vi "UNDTClasterToTbl.vi"(11 "UNDT_Cluster":T1 {"Gain Coeff" format="%#_6e"; "Reserve 1" format="%02x"; "Mux TX/RX" format="%02x"; "ScanDelay" format="%02x"; "PacketCounter" format="%08x"; "SamplingInterval" format="%#_6e"; "Lose Packet" format="%08x"; "EncodersParam2" format="%016x"; "EncodersParam1" format="%016x"; "CRC 8" format="%02x"; "N chanel" format="%02x"; "N tick" format="%02x"; "Ncycle" format="%04x"; "FrameFormatVersion" format="%02x"; "MagicWord" format="%.0x"}) -> (2 "appended array":string[](array[string]), 3 "Table Control":string[][](table))   [LabVIEW 2017]
uses:
  Control_EU/UNDT_ClusterPackRevers (Type).ctl
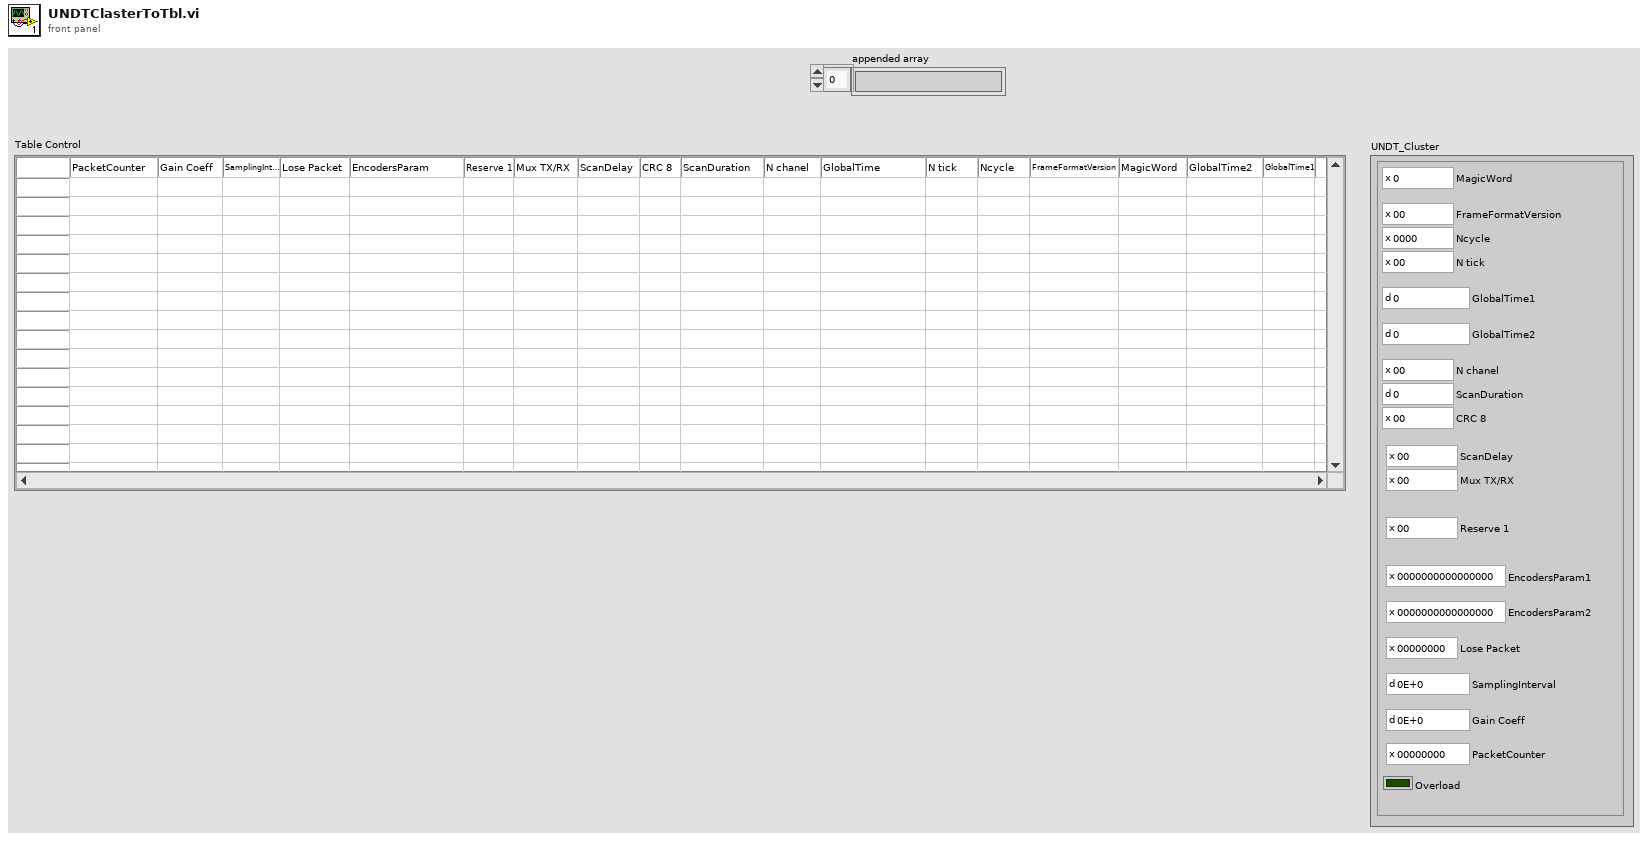
[diagram p1: front panel]
types:
  T1 = typedef "UNDT_ClusterPackRevers (Type).ctl" = cluster{"PacketCounter":u32, "Gain Coeff":sgl, "SamplingInterval":sgl, "Lose Packet":u32, "EncodersParam2":u64, "EncodersParam1":u64, "Reserve 1":u8, "Mux TX/RX":u8, "ScanDelay":u16, "CRC 8":u8, "ScanDuration":u16, "N chanel":u8, "GlobalTime2":u32, "GlobalTime1":u32, "N tick":u8, "Ncycle":u16, "FrameFormatVersion":u8, "MagicWord":u32, "Overload":bool}
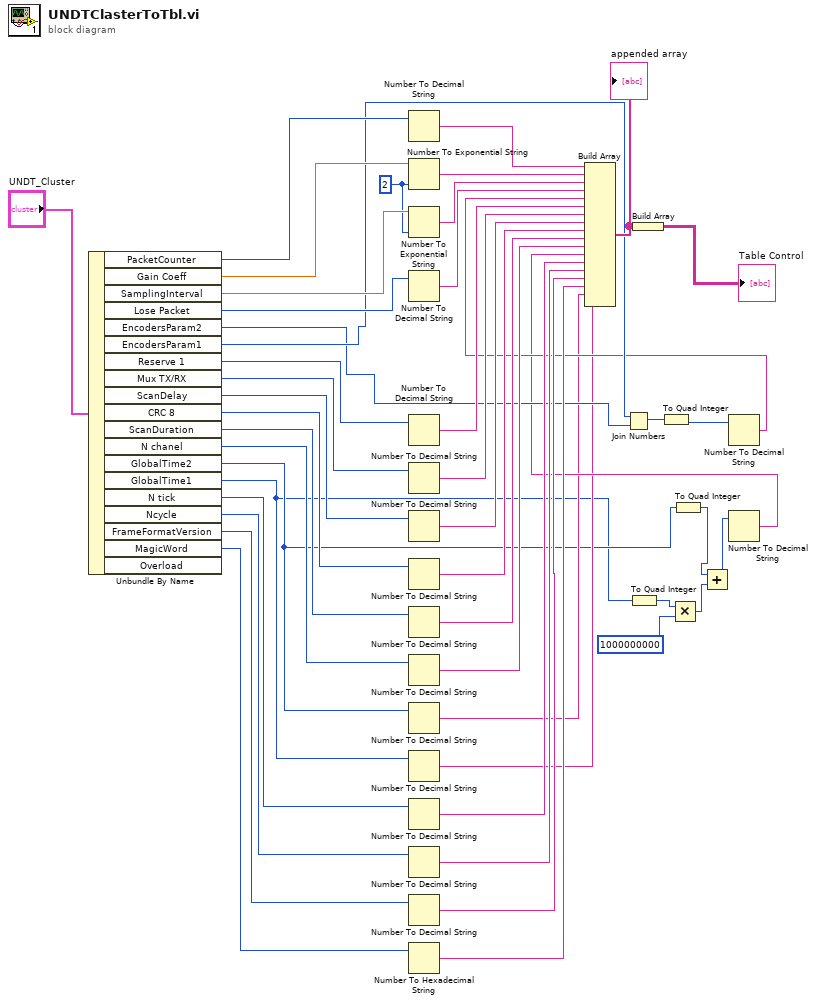
[diagram p0: block diagram]
diagram:
  w16 = i16 2 ("precision (6)")
  n1 = Unbundle By Name("UNDT_Cluster") -> ("PacketCounter"=w46:u32, "Gain Coeff"=w35:sgl, "SamplingInterval"=w19:sgl, "Lose Packet"=w18:u32, "EncodersParam2"=w14:u64, "EncodersParam1"=w15:u64, "Reserve 1"=w45:u8, "Mux TX/RX"=w44:u8, "ScanDelay"=w43:u16, "CRC 8"=w42:u8, "ScanDuration"=w41:u16, "N chanel"=w40:u8, "GlobalTime2"=w2:u32, "GlobalTime1"=w1:u32, "N tick"=w39:u8, "Ncycle"=w38:u16, "FrameFormatVersion"=w37:u8, "MagicWord"=w36:u32)  [unwired: 1 out]
  n2 = Number To Decimal String(number=w46) -> (decimal integer string=w34:string)  [unwired: 1 in]
  n3 = Number To Exponential String(number=w35, precision (6)=w16) -> (E-format string=w33:string)  [unwired: 2 in]
  n4 = Number To Exponential String(number=w19, precision (6)=w16) -> (E-format string=w32:string)  [unwired: 2 in]
  n5 = Number To Decimal String(number=w18) -> (decimal integer string=w17:string)  [unwired: 1 in]
  n6 = Number To Decimal String(number=w45) -> (decimal integer string=w31:string)  [unwired: 1 in]
  n7 = Number To Decimal String(number=w44) -> (decimal integer string=w30:string)  [unwired: 1 in]
  n8 = Number To Decimal String(number=w43) -> (decimal integer string=w29:string)  [unwired: 1 in]
  n9 = Number To Decimal String(number=w42) -> (decimal integer string=w28:string)  [unwired: 1 in]
  n10 = Number To Decimal String(number=w41) -> (decimal integer string=w27:string)  [unwired: 1 in]
  n11 = Number To Decimal String(number=w40) -> (decimal integer string=w26:string)  [unwired: 1 in]
  n12 = Number To Decimal String(number=w2) -> (decimal integer string=w9:string)  [unwired: 1 in]
  n13 = Number To Decimal String(number=w1) -> (decimal integer string=w8:string)  [unwired: 1 in]
  n14 = Number To Decimal String(number=w39) -> (decimal integer string=w25:string)  [unwired: 1 in]
  n15 = Number To Decimal String(number=w38) -> (decimal integer string=w24:string)  [unwired: 1 in]
  n16 = Number To Decimal String(number=w37) -> (decimal integer string=w23:string)  [unwired: 1 in]
  n17 = Number To Hexadecimal String(2:w36) -> (0:w22:string)  [unwired: 1 in]
  n18 = Join Numbers(hi=w15, lo=w14) -> ((hi.lo)=w13:u64)
  n19 = To Quad Integer(1:w1) -> (0:w7:i64)
  n20 = To Quad Integer(1:w13) -> (0:w12:i64)
  n21 = Multiply(x=w7, y=i64 1000000000) -> (x*y=w5:i64)
  n22 = To Quad Integer(1:w2) -> (0:w4:i64)
  n23 = Add(x=w4, y=w5) -> (x+y=w3:i64)
  n24 = Number To Decimal String(number=w12) -> (decimal integer string=w11:string)  [unwired: 1 in]
  n25 = Number To Decimal String(number=w3) -> (decimal integer string=w10:string)  [unwired: 1 in]
  n26 = Build Array(w34, w33, w32, w17, w11, w31, w30, w29, w28, w27, w26, w10, w25, w24, w23, w22, w9, w8) -> (w21:string[])
  "appended array" <- w21
  n27 = Build Array(w21) -> (→"Table Control":string[][])
